vi "RPC Get Driver Paths and Version.vi"(5 "Driver ID (\"\")":string, 7 "Driver Type (\"\")":string, 8 "error in (no error)":errorcluster, 10 "Base Path (empty)":path, 11 "app reference (empty)":refnum<vi>) -> (0 "error out":errorcluster, 1 "Driver Config Path":path, 2 "Driver Component Path":path, 3 "app reference":refnum<vi>, 4 "Component Version":cluster{"Version":string, "Build Number":u32}, 6 "version error?":bool)   [LabVIEW 2011]
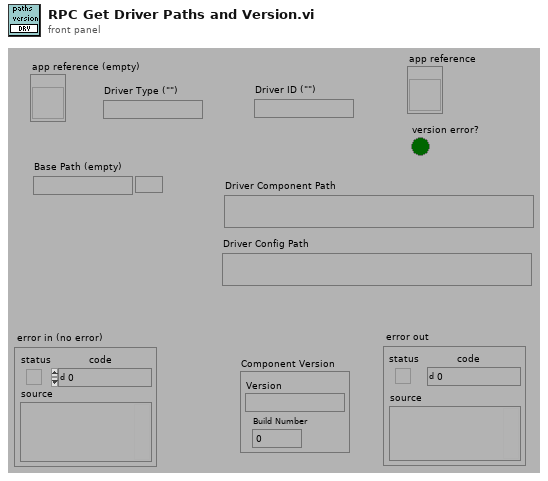
[diagram p1: front panel]
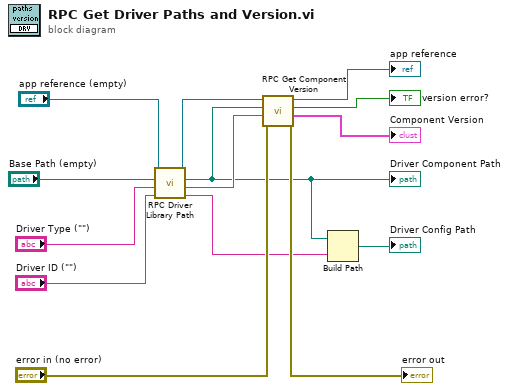
[diagram p0: block diagram]
diagram:
  n1 = call "RPC Driver Library Path.vi"("Driver ID (\"\")"="Driver ID (\"\")", "Driver Type (\"\")"="Driver Type (\"\")", "Base Path (empty)"="Base Path (empty)", "App Ref (null: local)"="app reference (empty)") -> ("Driver Config Name"=w5:string, "Driver Component Name"=w6:string, "Driver Library Path"=w2:path, "dup App Ref"=w3:refnum<vi>)  [unwired: 4 out]
  "Driver Component Path" <- w2
  n2 = call "RPC Get Component Version.vi"("error in (no error)"="error in (no error)", "Component (\"\")"=w6, "Component Library (empty)"=w2, "app reference (empty)"=w3) -> ("error out"=→"error out":errorcluster, "Component Version"=→"Component Version":cluster{"Version":string, "Build Number":u32}, "vi ref valid?"=→"version error?":bool, "app reference"=→"app reference":refnum<vi>)  [unwired: 4 out]
  n3 = Build Path(base path=w2, name or relative path=w5) -> (appended path=→"Driver Config Path":path)
